vi "Mean.vi"   [LabVIEW 2022 SP3, in "NI_AALBase.lvlib"]
uses:
  NI_AALBase.lvlib
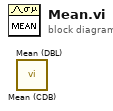
[diagram p0: block diagram]
diagram:
  n1 = call "Mean (CDB).vi"() -> ()  [unwired: 1 in, 2 out]
  n2 = call "Mean (DBL).vi"() -> ()  [unwired: 1 in, 2 out]
